vi "测试素数.vi"(11 "Num":i32=100) -> (3 "Prime":bool)   [LabVIEW 2013]
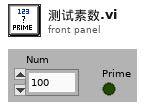
[diagram p1: front panel]
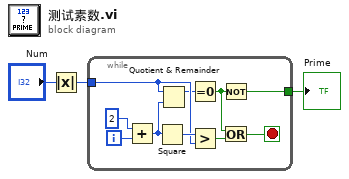
[diagram p0: block diagram]
diagram:
  n1 = Absolute Value(x="Num") -> (abs(x)=w2:i32)
  n2 = while {
    tunnel: w2 -> [w10]
    tunnel: [w4] -> w1
    i -> [w13]
    stop <- w7 stop-if-true
    n3 = Add(x=2, y=w13) -> (x+y=w9:i32)
    n4 = Square(x=w9) -> (x^2=w11:i32)
    n5 = Quotient & Remainder(x=w10, y=w9) -> (x-y*floor(x/y)=w8:i32)  [unwired: 1 out]
    n6 = Equal To 0?(x=w8) -> (x = 0?=w5:bool)
    n7 = Greater?(x=w11, y=w10) -> (0:w6:bool)
    n8 = Not(x=w5) -> (.not. x?=w4:bool)
    n9 = Or(x=w5, y=w6) -> (x .or. y?=w7:bool)
  }
  "Prime" <- w1
